vi "Continuous_Sound_Output_ph.vi"() -> ()   [LabVIEW 2022 SP3]
doc: "This VI demonstrates how to output continuous sound using SO Set Num Buffers. This example is available only on Windows."
uses:
  <vilib>/SOUND/lvsound.llb/Sound Format.ctl
  <vilib>/measure/NI_MABase.lvlib
panel:
  out "error out":errorcluster
  in  "Frequency":i32(slide)=440 scale=20.0..2000.0
  in  "stop":bool
  in  "Number of buffers":i32(slide)=1 scale=0.0..4.0
  # "Continuous Sound Output Using Buffers"
  # "This VI generates a sine tone using the Sound Output VIs.  It demonstrates the effect\nof SO Set Num Buffers.vi.  Setting \"Number of buffers\" to zero causes \"SO Wait.vi\" to\ncause  gaps in the sound.  Setting \"Number of buffers\" to one eliminates the gaps,\nbut you may still hear a gap if you switch windows or applications.  Setting \"Number\nof buffers\" even larger makes it less likely you will hear gaps, at the expense of more\nmemory and a larger delay between creating the data and actual sound generation."
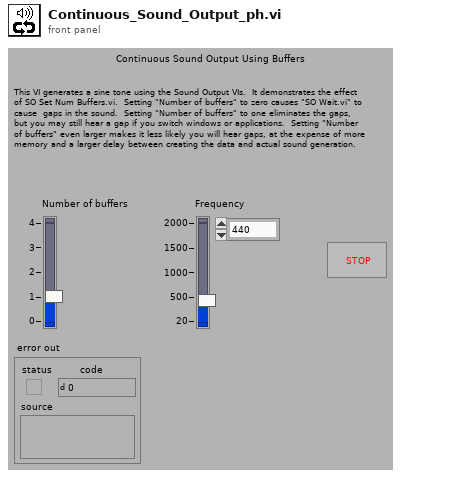
[diagram p1: front panel]
types:
  T1 = typedef "Sound Format.ctl" = cluster{"sound quality":enum16{"mono", "stereo"}, "rate":enum16{"11025", "22050", "44100", "8000"}, "bits per sample":enum16{"8 bit", "16 bit"}}
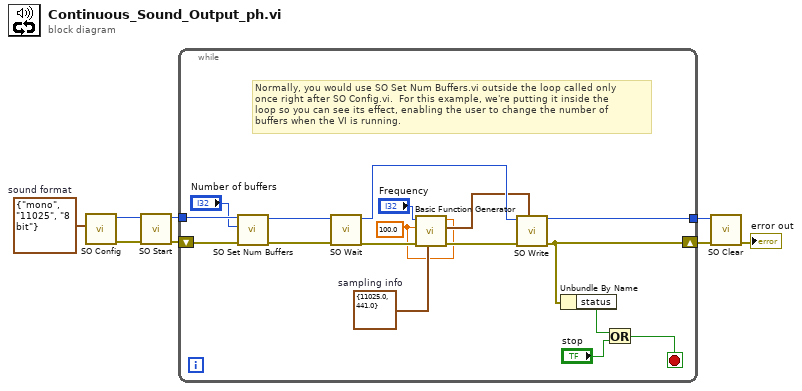
[diagram p0: block diagram]
diagram:
  w8 = T1 {"sound quality"=enum."mono", "rate"=enum."11025", "bits per sample"=enum."8 bit"}  # sound format
  n1 = call <vilib>:"SO Config.vi"("sound format"=w8) -> ("error out"=w6:errorcluster, "task ID out"=w7:u32)  [unwired: 1 in, 8 out]
  n2 = call <vilib>:"SO Start.vi"("error in (no error)"=w6, "task ID in"=w7) -> ("error out"=w5:errorcluster, "task ID out"=w4:u32)  [unwired: 8 out]
  n3 = while {
    shift-right: [w22] -> w3
    shift-left: w5 -> [w15]
    tunnel: w4 -> [w13]
    tunnel: [w10] -> w2
    stop <- w23 stop-if-true
    w17 = cluster{"Fs":dbl, "#s":dbl} {"Fs"=11025.0, "#s"=441.0}  # sampling info
    w9 = 100.0 ("amplitude")
    # "Normally, you would use SO Set Num Buffers.vi outside the loop called only\nonce right after SO Config.vi.  For this example, we're putting it inside the\nloop so you can see its effect, enabling the user to change the number of\nbuffers when the VI is running."
    n4 = call <vilib>:"SO Set Num Buffers.vi"("error in (no error)"=w15, "number of buffers"="Number of buffers", "task ID in"=w13) -> ("error out"=w14:errorcluster, "task ID out"=w12:u32)  [unwired: 7 out]
    n5 = call <vilib>:"SO Wait.vi"("error in (no error)"=w14, "task ID in"=w12) -> ("error out"=w20:errorcluster, "task ID out"=w25:u32)  [unwired: 8 out]
    n6 = call <vilib>:"Basic Function Generator.vi"("offset"=w9, "sampling info"=w17, "error in (no error)"=w20, "amplitude"=w9, "frequency"="Frequency") -> ("error out"=w19:errorcluster, "signal out"=w16:waveform(dbl))  [unwired: 4 in, 1 out]
    n7 = call <vilib>:"SO Write.vi"("mono 8-bit"=w16, "error in (no error)"=w19, "task ID in"=w25) -> ("error out"=w22:errorcluster, "task ID out"=w10:u32)  [unwired: 3 in, 4 out]
    n8 = Unbundle By Name(w22) -> ("status"=w21:bool)
    n9 = Or(x=w21, y="stop") -> (x .or. y?=w23:bool)
  }
  n10 = call <vilib>:"SO Clear.vi"("error in (no error)"=w3, "task ID in"=w2) -> ("error out"=→"error out":errorcluster)  [unwired: 9 out]
